vi "Fill_Combo_API_Box (SubVI).vi"(10 "configuration file path":path=path "D:/James Pratice LV/MQTT.ini", 11 "ComboBox in":refnum<vi>) -> ()   [LabVIEW 2018]
uses:
  <vilib>/Utility/miscctls.llb/LVComboBoxStrsAndValuesArrayTypeDef.ctl
  <vilib>/Utility/config.llb/Read Key (String).vi
  <vilib>/Utility/config.llb/NI_LVConfig.lvlib
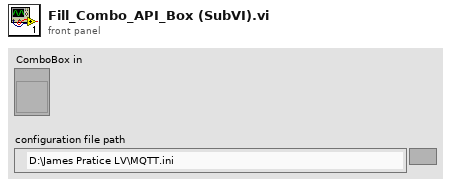
[diagram p1: front panel]
types:
  T1 = typedef "LVComboBoxStrsAndValuesArrayTypeDef.ctl" = cluster{"String":string, "Value":string}[]
  T2 = typedef "NI_LVConfig.lvlib/Config Data RefNum.ctl" = refnum<k1>
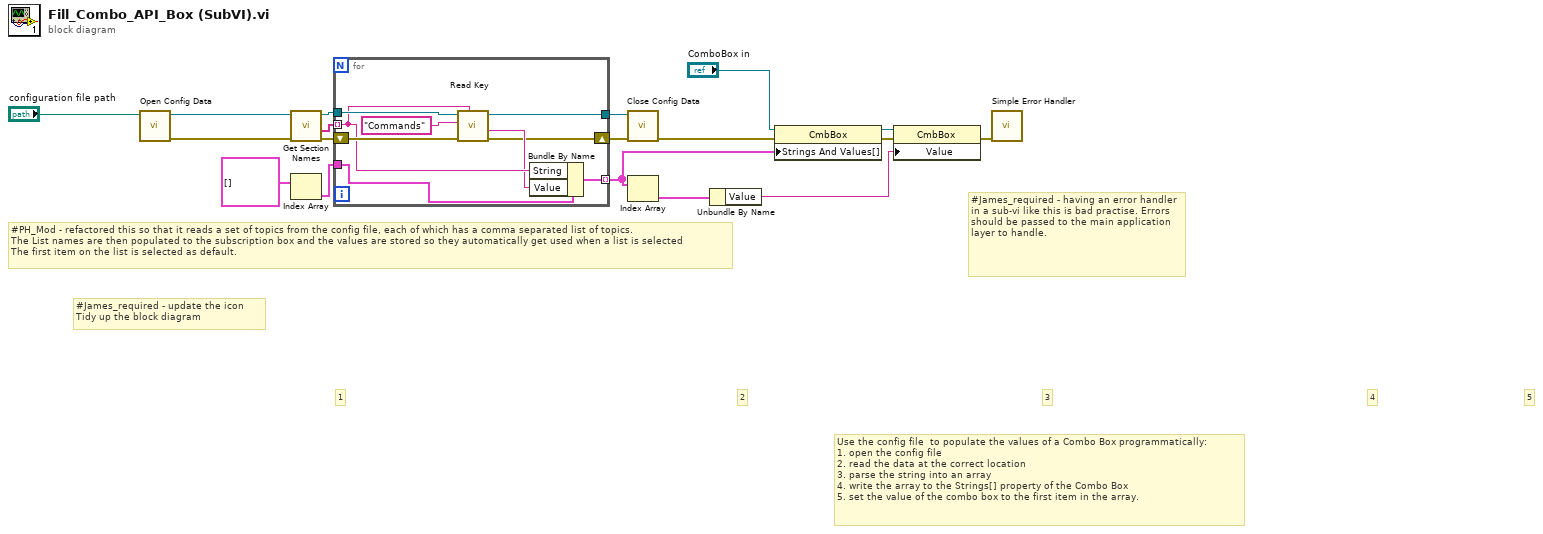
[diagram p0: block diagram]
diagram:
  # "#James_required - having an error handler in a sub-vi like this is bad practise. Errors should be passed to the main application layer to handle."
  # "#James_required - update the icon\nTidy up the block diagram"
  # "#PH_Mod - refactored this so that it reads a set of topics from the config file, each of which has a comma separated list of topics.\nThe List names are then populated to the subscription box and the values are stored so they automatically get used when a list is selected\nThe first item on the list is selected as default."
  # "5"
  # "4"
  # "3"
  # "2"
  # "1"
  # "Use the config file  to populate the values of a Combo Box programmatically:\n1. open the config file\n2. read the data at the correct location\n3. parse the string into an array\n4. write the array to the Strings[] property of the Combo Box\n5. set the value of the combo box to the first item in the array."
  n1 = call <vilib>:"Open Config Data.vi"("configuration file path"="configuration file path") -> ("error out"=w16:errorcluster, "refnum"=w14:T2)  [unwired: 8 in, 1 out]
  n2 = call <vilib>:"Get Section Names.vi"("error in (no error)"=w16, "refnum"=w14) -> ("error out"=w15:errorcluster, "section names"=w8:string[], "refnum out"=w13:T2)  [unwired: 7 in]
  n3 = Index Array(array=T1 [] ("Strings And Values []")) -> (element=w6:cluster{"String":string, "Value":string})  [unwired: 1 in]
  n4 = for {
    tunnel: w13 -> [w26]
    shift-right: [w19] -> w1
    shift-left: w15 -> [w27]
    tunnel: w8 -> [w23] mode=indexing
    tunnel: w6 -> [w24]
    tunnel: [w21] -> w5 mode=indexing
    tunnel: [w20] -> w3
    n5 = call-poly <vilib>:"Read Key.vi"("section"=w23, "error in (no error)"=w27, "key"="Commands", "refnum"=w26) -> ("error out"=w19:errorcluster, "value"=w22:string, "refnum out"=w20:T2)  [unwired: 4 in, 1 out]
    n6 = Bundle By Name(cluster=w24, "String"=w23, "Value"=w22) -> (w21:cluster{"String":string, "Value":string})
  }
  n7 = call <vilib>:"Close Config Data.vi"("error in (no error)"=w1, "refnum"=w3) -> ("error out"=w2:errorcluster)  [unwired: 8 in, 1 out]
  n8 = Index Array "Index Array"(array=w5) -> (element=w11:cluster{"String":string, "Value":string})  [unwired: 1 in]
  n9 = Unbundle By Name(w11) -> ("Value"=w4:string)
  n10 = property on="Property Node" class="CmbBox"(reference="ComboBox in", error in=w2, "Strings And Values[]"=w5) -> (reference out=w9:refnum<vi>, error out=w12:errorcluster)
  n11 = property on="Property Node" class="CmbBox"(reference=w9, error in=w12, "Value"=w4) -> (error out=w17:errorcluster)  [unwired: 1 out]
  n12 = call <vilib>:"Simple Error Handler.vi"("error in (no error)"=w17) -> ()  [unwired: 4 in, 5 out]
